vi "dfd_Halfband Design with Order.vi"(4 "fs in [Hz]":dbl=1.0 format="%#_2g", 5 "method":u16(ring)=3 items=["Kaiser Window", "Dolph-Chebyshev Window", "Equi-Ripple", "Positive Equi-Ripple", "Max Flat"], 6 "filtering mode":T1=2 items=["No Rate Change", "Interpolation", "Decimation"], 7 "filter type":enum16{"Lowpass", "Highpass"}(ring), 8 "error in (no error)":errorcluster, 10 "roll off":dbl=0.2, 11 "order":i32=20) -> (0 "error out":errorcluster, 2 "order out":i32, 3 "multirate filter out":T2={"mMRate_Structure"=enum."CIC", "mMRate_Mode"=0, "mMRate_Factor"=1, "mMRate_FIRParams"={"mMRate_FIR_H"=[], "mMRate_FIR_IsNyquist?"=FALSE, "mMRate_FIR_IsSymmetric?"=FALSE}, "mMRate_CICParams"={"mMRate_CIC_#Stage"=2, "mMRate_CIC_Lag"=1, "mMRate_CIC_Type"=enum."Lowpass"}, "mMRate_Order"=1, "mMRate_Version"="1.0", "mMRate_Comments"="1.0", "mMRate_RationalFactor"={"mMRate_L"=-1, "mMRate_M"=-1}, "mMRate_Fs"=1.0, "mMRate_Quantized?"=FALSE, "mMRate_QFilterGain"=1.0, "mMRate_CoefWl"=16, "mMRate_Scaling"={"mMRate_ScaleByPowerOf2?"=FALSE, "mMRate_ScaleType"=enum."Time Domain 1-Norm"}, "mMRate_InputWl"=0, "mMRate_OutputWl"=0, "mMRate_OutputMode"=enum."Nearest", "mMRate_MultMode"=enum."Truncated", "mMRate_BitPruning"=FALSE, "mMRate_GainWl"=16, "mMRate_OutputFwl"=0, "mMRate_SumIwl"=0, "mMRate_InputIwl "=16, "mMRate_SumWl"=32, "mMRate_CoefIwl"=0} {"mMRate_SumWl" min=1 max=32 step=1; "mMRate_InputIwl" min=1 max=32 step=1; "mMRate_GainWl" min=1 max=32 step=1; "mMRate_OutputWl" min=1 max=32 step=1; "mMRate_InputWl" min=1 max=32 step=1; "mMRate_CoefWl" min=1 max=32 step=1; "mMRate_Mode" items=["Default"=-1, "No Rate Change"=0, "Interpolation"=1, "Decimation"=2, "Interpolated"=3, "Rational"=4]})   [LabVIEW 2017, in "NI_DigFilterLicensed.lvlib"]
doc: "Designs a halfband FIR filter with order specified. The filter can be used as a normal filter, an interpolator or a decimator."
uses:
  <vilib>/addons/Digital Filter Design/NI_DigFilterLicensed.lvlib
  <vilib>/addons/Digital Filter Design/_Objects.llb/DFD Multirate Filter Obj.ctl
  <vilib>/addons/Digital Filter Design/_Objects.llb/DFD Multirate Mode.ctl
  <vilib>/addons/Digital Filter Design/_Objects.llb/DFD Coef Norm Type.ctl
  <vilib>/addons/Digital Filter Design/_Objects.llb/DFD Round-off Mode.ctl
  <vilib>/addons/Digital Filter Design/_Objects.llb/DFD FXP MRate Multiply Mode.ctl
  <vilib>/addons/Digital Filter Design/_Objects.llb/DFD Multirate Filtering Mode.ctl
  <vilib>/addons/Digital Filter Design/FilterLib.llb/DFD Build MRate Filter from TF.vi
  <vilib>/addons/Digital Filter Design/NI_DigFilter_Process.lvlib
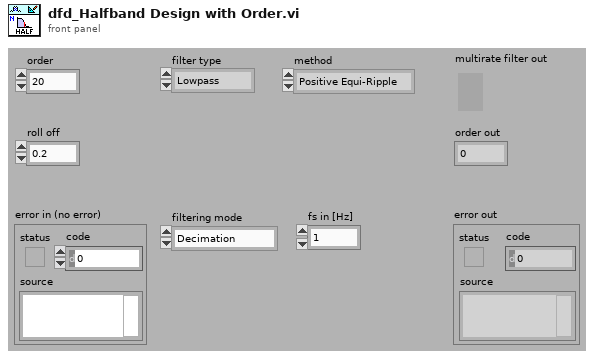
[diagram p1: front panel]
types:
  T1 = typedef "NI_DigFilterLicensed.lvlib/DFD Multirate Filtering Mode.ctl" = u16
  T2 = typedef "NI_DigFilterLicensed.lvlib/DFD Multirate Filter Obj.ctl" = cluster{"mMRate_Structure":enum16{"CIC", "FIR", "IIR", "Lattice"}, "mMRate_Mode":T3, "mMRate_Factor":i32, "mMRate_FIRParams":cluster{"mMRate_FIR_H":dbl[], "mMRate_FIR_IsNyquist?":bool, "mMRate_FIR_IsSymmetric?":bool}, "mMRate_CICParams":cluster{"mMRate_CIC_#Stage":i32, "mMRate_CIC_Lag":i32, "mMRate_CIC_Type":enum16{"Lowpass", "Highpass"}}, "mMRate_Order":i32, "mMRate_Version":string, "mMRate_Comments":string, "mMRate_RationalFactor":cluster{"mMRate_L":i32, "mMRate_M":i32}, "mMRate_Fs":dbl, "mMRate_Quantized?":bool, "mMRate_QFilterGain":dbl, "mMRate_CoefWl":i16, "mMRate_Scaling":cluster{"mMRate_ScaleByPowerOf2?":bool, "mMRate_ScaleType":T4}, "mMRate_InputWl":i16, "mMRate_OutputWl":i16, "mMRate_OutputMode":T5, "mMRate_MultMode":T6, "mMRate_BitPruning":bool, "mMRate_GainWl":i16, "mMRate_OutputFwl":i16, "mMRate_SumIwl":i16, "mMRate_InputIwl ":i16, "mMRate_SumWl":i16, "mMRate_CoefIwl":i16}
  T3 = typedef "NI_DigFilterLicensed.lvlib/DFD Multirate Mode.ctl" = i16
  T4 = typedef "NI_DigFilterLicensed.lvlib/DFD Coef Norm Type.ctl" = enum16{"No Norm", "Time Domain 1-Norm", "Time Domain 2-Norm", "Time Domain Inf-Norm"}
  T5 = typedef "NI_DigFilterLicensed.lvlib/DFD Round-off Mode.ctl" = enum16{"Nearest", "Truncation"}
  T6 = typedef "NI_DigFilterLicensed.lvlib/DFD FXP MRate Multiply Mode.ctl" = enum16{"Truncated", "Full"}
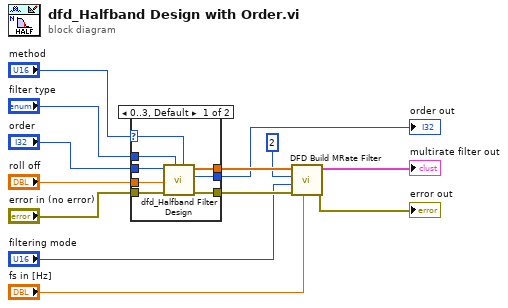
[diagram p0: block diagram]
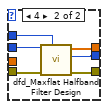
[diagram p2: hidden frame]
diagram:
  n1 = case shown="0..3, Default" "method" {
    selector: "method" -> [w14 _]
    tunnel: "filter type" -> [w21 w25]
    tunnel: "error in (no error)" -> [w20 w26]
    tunnel: "order" -> [w19 w27]
    tunnel: "roll off" -> [w18 _]
    tunnel: [w17 w23] -> w7
    tunnel: [w16 w22] -> w6
    tunnel: [w15 w24] -> w4
    frame 0..3, Default {
      n2 = call <vilib>:"dfd_Halfband Filter Design.vi"("method"=w14, "filter type"=w21, "error IO"=w20, "roll off"=w18, "order"=w19) -> ("error out"=w16:errorcluster, "order out"=w15:i32, "h out"=w17:dbl[])  [unwired: 4 out]
    }
    frame 4 {
      n3 = call <vilib>:"dfd_Maxflat Halfband Filter Design.vi"("filter type"=w25, "error IO"=w26, "order"=w27) -> ("error out"=w22:errorcluster, "order out"=w24:i32, "h out"=w23:dbl[])  [unwired: 6 out]
    }
  }
  "order out" <- w4
  n4 = call-poly <vilib>:"DFD Build MRate Filter.vi"("fs in [Hz]"="fs in [Hz]", "error in (no error)"=w6, "filtering mode"="filtering mode", "factor"=2, "h(n)"=w7) -> ("error out"=→"error out":errorcluster, "multirate filter out"=→"multirate filter out":T2)  [unwired: 5 out]
